vi "test Error Clusters Automatic Error Handling.vi"(8 "error in (no error)":errorcluster, 11 "TestCase in":refnum<class "Data Structure Tests.lvclass">) -> (0 "error out":errorcluster, 3 "TestCase out":refnum<class "Data Structure Tests.lvclass">)   [LabVIEW 2020, in "Data Structure Tests.lvclass"]
uses:
  Data Structure Tests.lvclass
  <vilib>/Utility/file.llb/Application Directory.vi
  <vilib>/Utility/libraryn.llb/Check if File or Folder Exists.vi
  <vilib>/addons/_JKI Toolkits/VI Tester/TestCase.llb/TestCase.lvclass
  C:/Program Files/National Instruments/LabVIEW 2024/vi.lib/addons/_JKI Toolkits/VI Tester/TestCase.llb/TestCase.lvclass
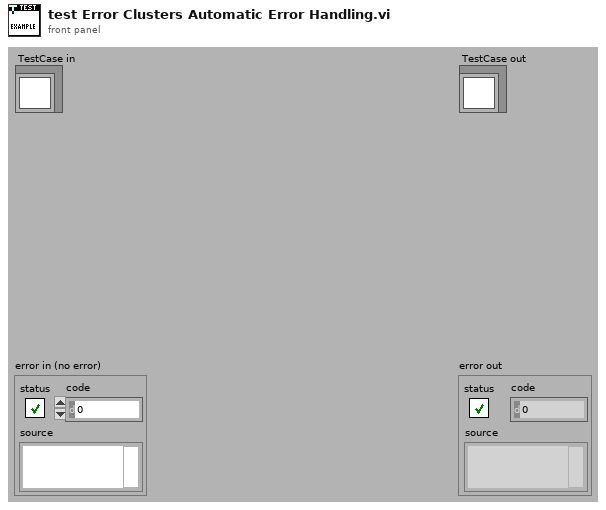
[diagram p1: front panel]
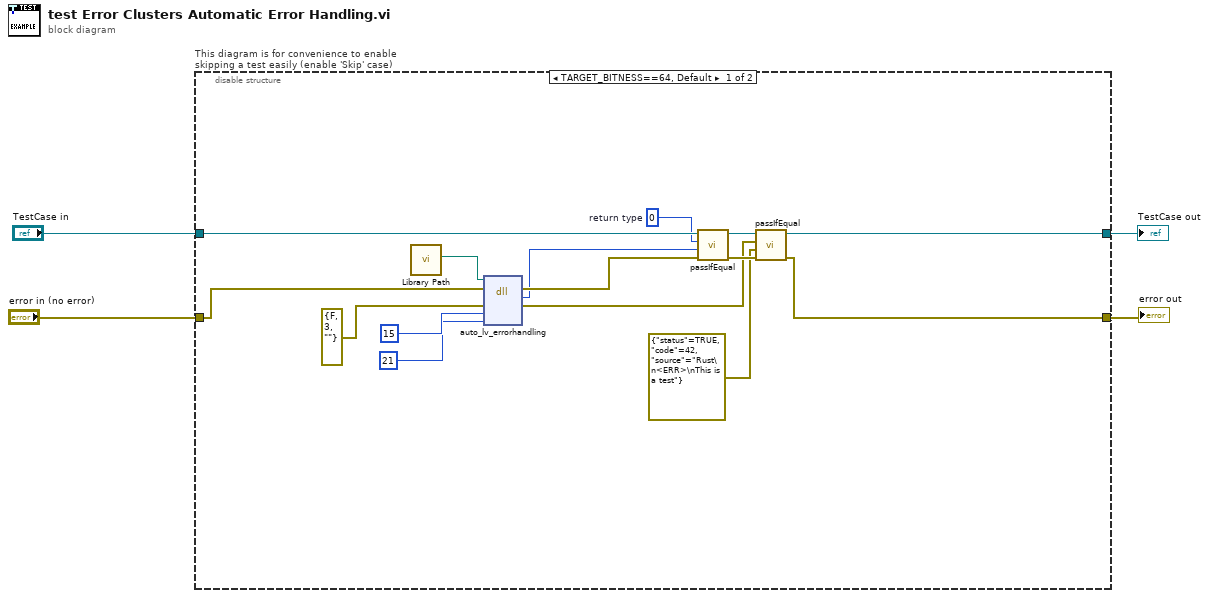
[diagram p0: block diagram]
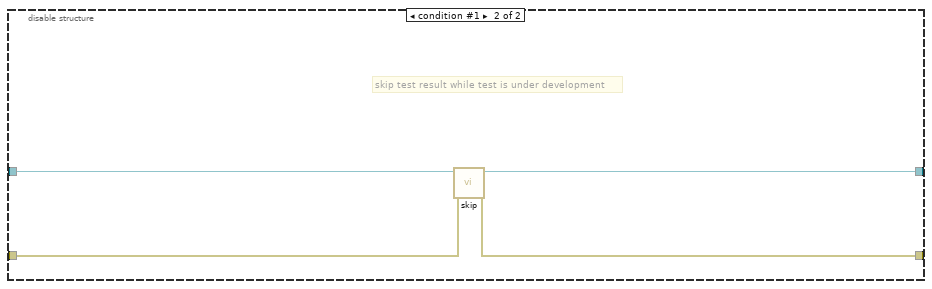
[diagram p2: hidden frame]
diagram:
  n1 = disable-structure "This diagram is for convenience to enable skipping a test easily (enable 'Skip' case)" shown="TARGET_BITNESS==64, Default" {
    disable-tunnel: "TestCase in" -> [w19 w23]
    disable-tunnel: [w13 w21] -> w1
    disable-tunnel: [w15 w22] -> w3
    disable-tunnel: "error in (no error)" -> [w17 w20]
    frame condition #0 (active) {
      w10 = 0  # return type
      n2 = call "Library Path.vi"() -> ("Library Path"=w12:path)  [unwired: 11 in]
      n3 = dll-call lib="C:/Users/JamesMcNally/Documents/RustInterop/Rust-LabVIEW-Interop/target/debug/labview_test_library.dll" fn="auto_lv_errorhandling"(path in=w12, error in=w17, "cluster"=errorcluster {"status"=FALSE, "code"=3, "source"=""} ("error constant"), "arg1"=15, "arg2"=21) -> (error out=w16:errorcluster, "return type"=w11:i32, "cluster"=w8:errorcluster)  [unwired: 3 in, 1 out]
      n4 = call-dynamic "passIfEqual.vi"("error in (no error)"=w16, "y"=w11, "x"=w10, "TestCase in"=w19) -> ("error out"=w18:errorcluster, "TestCase out"=w14:refnum<class "Data Structure Tests.lvclass">)  [unwired: 6 in]
      n5 = call-dynamic "passIfEqual.vi"("error in (no error)"=w18, "y"=errorcluster {"status"=TRUE, "code"=42, "source"="Rust\n<ERR>\nThis is a test"} ("error constant"), "x"=w8, "TestCase in"=w14) -> ("error out"=w15:errorcluster, "TestCase out"=w13:refnum<class "Data Structure Tests.lvclass">)  [unwired: 6 in]
    }
    frame condition #1 {
      # "skip test result while test is under development"
      n6 = call <vilib>:"skip.vi"("error in (no error)"=w20, "TestCase in"=w23) -> ("error out"=w22:errorcluster, "TestCase out"=w21:refnum<class "Data Structure Tests.lvclass">)  [unwired: 8 in]
    }
  }
  "error out" <- w3
  "TestCase out" <- w1
